vi "Fetch All Noise Measurement.vi"(0 "VISA resource name":refnum<visa-resource-name>, 5 "Query Level (0: Zero)":i32(ring) items=["Zero", "One"], 11 "error in (no error)":errorcluster) -> (1 "TI":T2, 2 "RN":T2, 3 "DI":T2, 4 "VISA resource name out":refnum<visa-resource-name>, 6 "ISI":T2, 8 "Misc":T1, 12 "PI":T3, 13 "ABUI":T2, 14 "BUI":T2, 15 "error out":errorcluster)   [LabVIEW 2020, in "Agilent 90000 Series.lvlib"]
doc: "Returns the noise measurement results for the specified level.\n\nNotes:\nThis VI does not check the instrument status. Typically, you call this VI only in a sequence of calls to other low-level driver VIs. The sequence performs one operation. You use the low-level VIs to optimize one or more aspects of interaction with the instrument. If you want to check the instrument status, call the Error-Query VI at the conclusion of the sequence."
uses:
  Agilent 90000 Series.lvlib
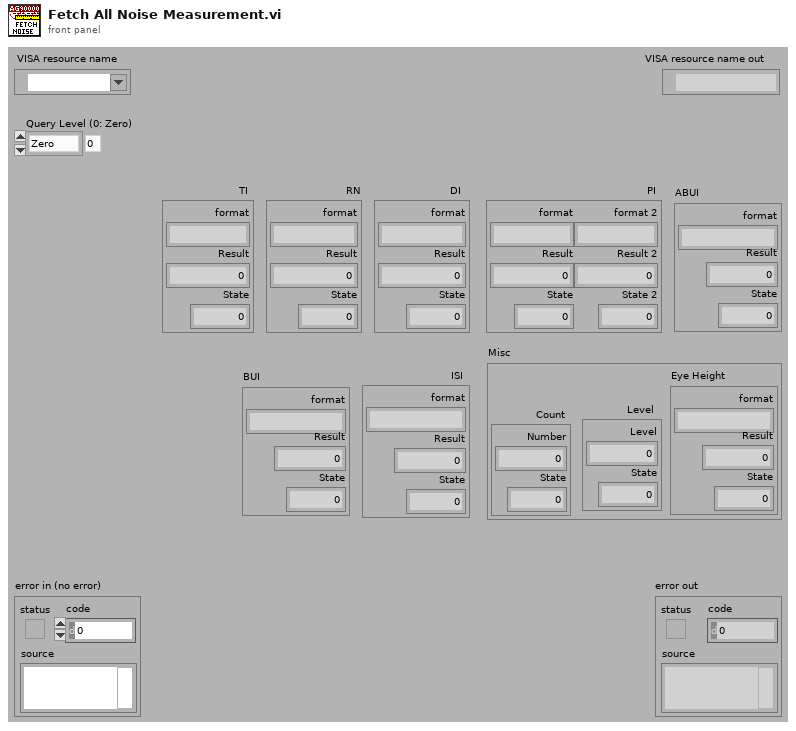
[diagram p1: front panel]
types:
  T1 = cluster{"Count":cluster{"Number":dbl, "State":i32}, "Level":cluster{"Level":dbl, "State":i32}, "Eye Height":cluster{"format":string, "Result":dbl, "State":i32}}
  T2 = cluster{"format":string, "Result":dbl, "State":i32}
  T3 = cluster{"format":string, "Result":dbl, "State":i32, "format 2":string, "Result 2":dbl, "State 2":i32}
  T4 = cluster{cluster{dbl, i32}, cluster{dbl, i32}, cluster{string, dbl, i32}}
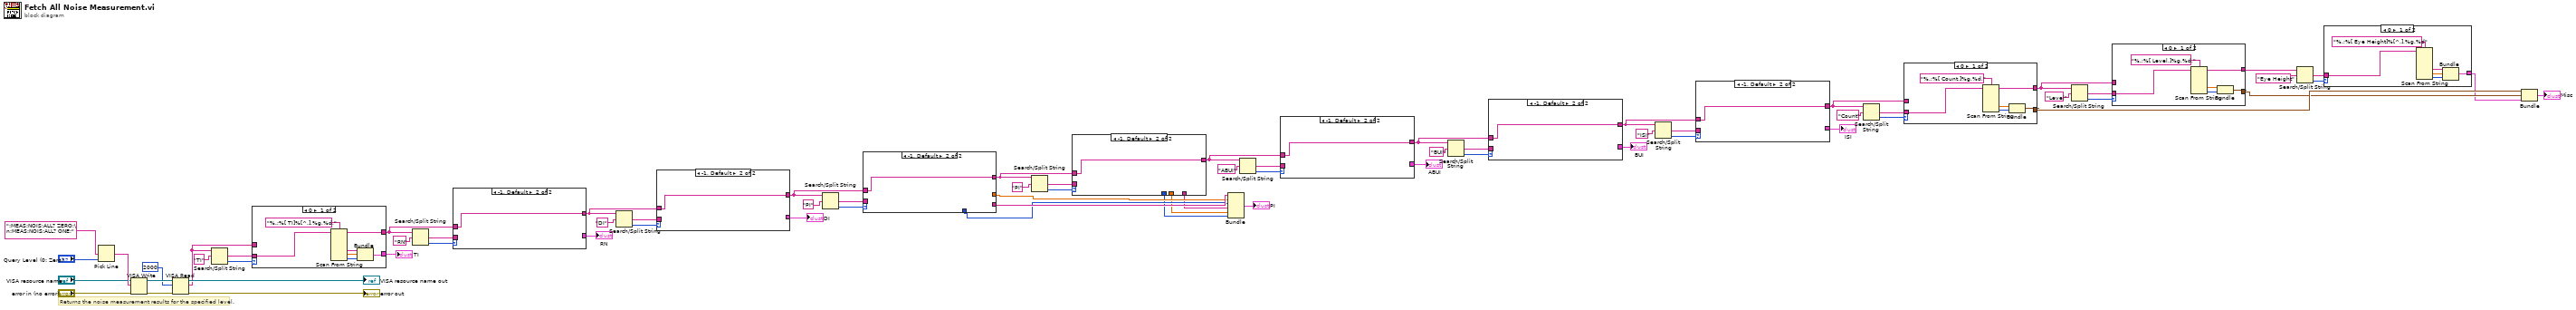
[diagram p0: block diagram]
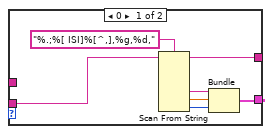
[diagram p5: hidden frame]
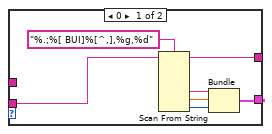
[diagram p6: hidden frame]
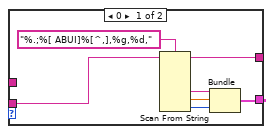
[diagram p7: hidden frame]
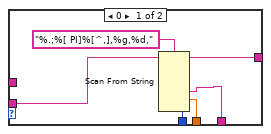
[diagram p8: hidden frame]
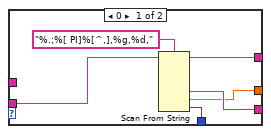
[diagram p9: hidden frame]
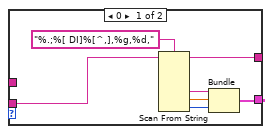
[diagram p10: hidden frame]
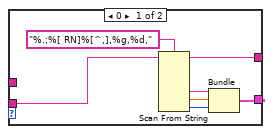
[diagram p11: hidden frame]
diagram:
  # "Returns the noise measurement results for the specified level."
  n1 = Pick Line(multi-line string=":MEAS:NOIS:ALL? ZERO;\n:MEAS:NOIS:ALL? ONE;", line index="Query Level (0: Zero)") -> (output string=w69:string)  [unwired: 1 out]
  n2 = VISA Write(VISA resource name="VISA resource name", write buffer=w69, error in (no error)="error in (no error)") -> (VISA resource name out=w65:refnum<visa-resource-name>, error out=w64:errorcluster)  [unwired: 1 out]
  n3 = VISA Read(VISA resource name=w65, byte count=u32 2000, error in (no error)=w64) -> (VISA resource name out=→"VISA resource name out":refnum<visa-resource-name>, read buffer=w58:string, error out=→"error out":errorcluster)  [unwired: 1 out]
  n4 = Search/Split String(string=w58, search string/char (-)="TI") -> (match + rest of string=w59:string, offset of match=w56:i32)  [unwired: 1 in, 1 out]
  n5 = case shown="0" w56 {
    tunnel: w59 -> [w74 _]
    tunnel: w58 -> [_ w79]
    tunnel: [w72 w79] -> w52
    tunnel: [w73 _] -> w57
    frame 0 {
      n6 = Scan From String(format string="%.;%[ TI]%[^,],%g,%d,", input string=w74) -> (remaining string=w72:string, output 2=w76:string, output 3=w77:dbl, output 4=w78:i32)  [unwired: 2 in, 7 out]
      n7 = Bundle(w76, w77, w78) -> (w73:cluster{string, dbl, i32})  [unwired: 1 out]
    }
    frame -1, Default {
    }
  }
  "TI" <- w57
  n8 = Search/Split String(string=w52, search string/char (-)="RN") -> (match + rest of string=w54:string, offset of match=w55:i32)  [unwired: 1 in, 1 out]
  n9 = case shown="-1, Default" w55 {
    tunnel: w54 -> [w82 _]
    tunnel: w52 -> [_ w87]
    tunnel: [w80 w87] -> w47
    tunnel: [w81 _] -> w51
    frame 0 {
      n10 = Scan From String(format string="%.;%[ RN]%[^,],%g,%d,", input string=w82) -> (remaining string=w80:string, output 2=w84:string, output 3=w85:dbl, output 4=w86:i32)  [unwired: 2 in, 7 out]
      n11 = Bundle(w84, w85, w86) -> (w81:cluster{string, dbl, i32})  [unwired: 1 out]
    }
    frame -1, Default {
    }
  }
  "RN" <- w51
  n12 = Search/Split String(string=w47, search string/char (-)="DI") -> (match + rest of string=w49:string, offset of match=w48:i32)  [unwired: 1 in, 1 out]
  n13 = case shown="-1, Default" w48 {
    tunnel: w49 -> [w90 _]
    tunnel: w47 -> [_ w95]
    tunnel: [w88 w95] -> w24
    tunnel: [w89 _] -> w46
    frame 0 {
      n14 = Scan From String(format string="%.;%[ DI]%[^,],%g,%d,", input string=w90) -> (remaining string=w88:string, output 2=w92:string, output 3=w93:dbl, output 4=w94:i32)  [unwired: 2 in, 7 out]
      n15 = Bundle(w92, w93, w94) -> (w89:cluster{string, dbl, i32})  [unwired: 1 out]
    }
    frame -1, Default {
    }
  }
  "DI" <- w46
  n16 = Search/Split String(string=w24, search string/char (-)="PI") -> (match + rest of string=w44:string, offset of match=w45:i32)  [unwired: 1 in, 1 out]
  n17 = case shown="-1, Default" w45 {
    tunnel: w44 -> [w100 _]
    tunnel: w24 -> [_ w102]
    tunnel: [w99 w102] -> w23
    tunnel: [w98 _] -> w13
    tunnel: [w97 _] -> w12
    tunnel: [w96 _] -> w11
    frame 0 {
      n18 = Scan From String(format string="%.;%[ PI]%[^,],%g,%d,", input string=w100) -> (remaining string=w99:string, output 2=w98:string, output 3=w97:dbl, output 4=w96:i32)  [unwired: 2 in, 7 out]
    }
    frame -1, Default {
    }
  }
  n19 = Search/Split String(string=w23, search string/char (-)="PI") -> (match + rest of string=w41:string, offset of match=w40:i32)  [unwired: 1 in, 1 out]
  n20 = case shown="-1, Default" w40 {
    tunnel: w41 -> [w107 _]
    tunnel: w23 -> [_ w109]
    tunnel: [w106 w109] -> w19
    tunnel: [w105 _] -> w10
    tunnel: [w104 _] -> w9
    tunnel: [w103 _] -> w8
    frame 0 {
      n21 = Scan From String(format string="%.;%[ PI]%[^,],%g,%d,", input string=w107) -> (remaining string=w106:string, output 2=w105:string, output 3=w104:dbl, output 4=w103:i32)  [unwired: 2 in, 7 out]
    }
    frame -1, Default {
    }
  }
  n22 = Bundle(w13, w12, w11, w10, w9, w8) -> (→"PI":cluster{string, dbl, i32, string, dbl, i32})  [unwired: 1 out]
  n23 = Search/Split String(string=w19, search string/char (-)="ABUI") -> (match + rest of string=w38:string, offset of match=w39:i32)  [unwired: 1 in, 1 out]
  n24 = case shown="-1, Default" w39 {
    tunnel: w38 -> [w112 _]
    tunnel: w19 -> [_ w117]
    tunnel: [w110 w117] -> w18
    tunnel: [w111 _] -> w7
    frame 0 {
      n25 = Scan From String(format string="%.;%[ ABUI]%[^,],%g,%d,", input string=w112) -> (remaining string=w110:string, output 2=w114:string, output 3=w115:dbl, output 4=w116:i32)  [unwired: 2 in, 7 out]
      n26 = Bundle(w114, w115, w116) -> (w111:cluster{string, dbl, i32})  [unwired: 1 out]
    }
    frame -1, Default {
    }
  }
  "ABUI" <- w7
  n27 = Search/Split String(string=w18, search string/char (-)="BUI") -> (match + rest of string=w35:string, offset of match=w34:i32)  [unwired: 1 in, 1 out]
  n28 = case shown="-1, Default" w34 {
    tunnel: w35 -> [w120 _]
    tunnel: w18 -> [_ w125]
    tunnel: [w118 w125] -> w17
    tunnel: [w119 _] -> w6
    frame 0 {
      n29 = Scan From String(format string="%.;%[ BUI]%[^,],%g,%d", input string=w120) -> (remaining string=w118:string, output 2=w122:string, output 3=w123:dbl, output 4=w124:i32)  [unwired: 2 in, 7 out]
      n30 = Bundle(w122, w123, w124) -> (w119:cluster{string, dbl, i32})  [unwired: 1 out]
    }
    frame -1, Default {
    }
  }
  "BUI" <- w6
  n31 = Search/Split String(string=w17, search string/char (-)="ISI") -> (match + rest of string=w32:string, offset of match=w33:i32)  [unwired: 1 in, 1 out]
  n32 = case shown="-1, Default" w33 {
    tunnel: w32 -> [w128 _]
    tunnel: w17 -> [_ w133]
    tunnel: [w126 w133] -> w16
    tunnel: [w127 _] -> w5
    frame 0 {
      n33 = Scan From String(format string="%.;%[ ISI]%[^,],%g,%d,", input string=w128) -> (remaining string=w126:string, output 2=w130:string, output 3=w131:dbl, output 4=w132:i32)  [unwired: 2 in, 7 out]
      n34 = Bundle(w130, w131, w132) -> (w127:cluster{string, dbl, i32})  [unwired: 1 out]
    }
    frame -1, Default {
    }
  }
  "ISI" <- w5
  n35 = Search/Split String(string=w16, search string/char (-)="Count") -> (match + rest of string=w29:string, offset of match=w28:i32)  [unwired: 1 in, 1 out]
  n36 = case shown="0" w28 {
    tunnel: w29 -> [w136 _]
    tunnel: w16 -> [_ w140]
    tunnel: [w134 w140] -> w15
    tunnel: [w135 _] -> w4
    frame 0 {
      n37 = Scan From String(format string="%.;%[ Count,]%g,%d,", input string=w136) -> (remaining string=w134:string, output 2=w138:dbl, output 3=w139:i32)  [unwired: 2 in, 6 out]
      n38 = Bundle(w138, w139) -> (w135:cluster{dbl, i32})  [unwired: 1 out]
    }
    frame -1, Default {
    }
  }
  n39 = Search/Split String(string=w15, search string/char (-)="Level") -> (match + rest of string=w26:string, offset of match=w27:i32)  [unwired: 1 in, 1 out]
  n40 = case shown="0" w27 {
    tunnel: w26 -> [w143 _]
    tunnel: w15 -> [_ w147]
    tunnel: [w141 w147] -> w14
    tunnel: [w142 _] -> w3
    frame 0 {
      n41 = Scan From String(format string="%.;%[ Level,]%g,%d,", input string=w143) -> (remaining string=w141:string, output 2=w145:dbl, output 3=w146:i32)  [unwired: 2 in, 6 out]
      n42 = Bundle(w145, w146) -> (w142:cluster{dbl, i32})  [unwired: 1 out]
    }
    frame -1, Default {
    }
  }
  n43 = Search/Split String(string=w14, search string/char (-)="Eye Height") -> (match + rest of string=w21:string, offset of match=w20:i32)  [unwired: 1 in, 1 out]
  n44 = case shown="0" w20 {
    tunnel: w21 -> [w149 _]
    tunnel: [w148 _] -> w2
    frame 0 {
      n45 = Scan From String(format string="%.;%[ Eye Height]%[^,],%g,%d", input string=w149) -> (output 2=w151:string, output 3=w152:dbl, output 4=w153:i32)  [unwired: 2 in, 8 out]
      n46 = Bundle(w151, w152, w153) -> (w148:cluster{string, dbl, i32})  [unwired: 1 out]
    }
    frame -1, Default {
    }
  }
  n47 = Bundle(w4, w3, w2) -> (→"Misc":T4)  [unwired: 1 out]
